vi "12.2-3 ParticleRemove.vi"() -> ()   [LabVIEW 2016]
doc: "This example shows how to use the Edge Tool in NI Vision. The Edge Tool finds edges (or sharp transitions in the pixels values) along a given line or ROI profile. The Edge Tool is a precursor function to many of the gauging and inspection tasks. For example, the location of the edges found along a line profile across an object can interpreted as the boundaries of the object whose dimensions have to be measured for a gauging application or the presence of a crack in the surface of an object for an inspection application."
uses:
  <vilib>/vision/NI_Vision_Development_Module.lvlib
panel:
  in  "Connectivity":bool
  in  "Filter":bool
  out "Src":T1(plugin-control)
  in  "Hexa Pixel?":bool
  in  "# of iterations":i32=20
  out "Dst":T1(plugin-control)
  in  "Stop":bool
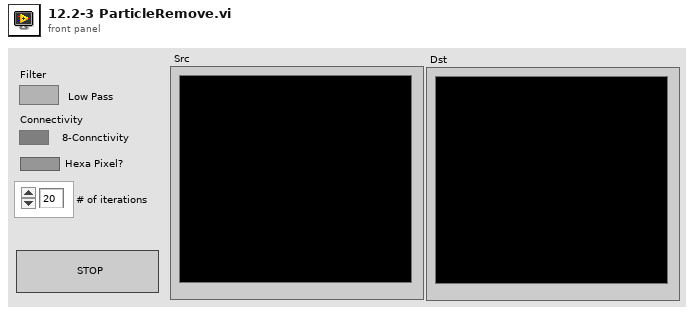
[diagram p1: front panel]
types:
  T1 = typedef "IMAQ Image.ctl" = refnum<image>
  T2 = cluster{"Connectivity":bool, "Hexa Pixel?":bool, "# of iterations":i32, "Filter":bool}
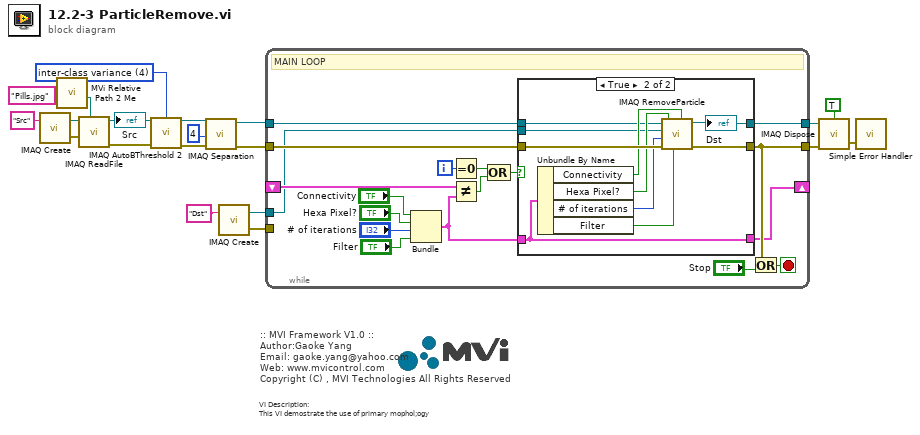
[diagram p0: block diagram]
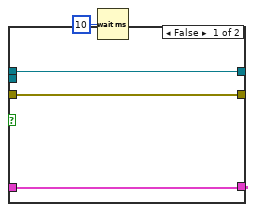
[diagram p2: hidden frame]
diagram:
  w9 = 4 items=["clustering", "entropy", "metric", "moments", "inter-class variance"] ("Method")
  # "VI Description:\nThis VI demostrate the use of primary mophol;ogy"
  # ":: MVI Framework V1.0 ::\nAuthor:Gaoke Yang\nEmail: gaoke.yang@yahoo.com\nWeb: www.mvicontrol.com\nCopyright (C) , MVI Technologies All Rights Reserved"
  n1 = call "IMAQ Create"("Image Name"="Src") -> ("New Image"=w19:T1, "error out"=w18:errorcluster)  [unwired: 4 in]
  n2 = call "MVi Relative Path 2 Me.vi"("Relative Path"="Pills.jpg" ("name or relative path")) -> ("Appended Dir"=w14:path)  [unwired: 5 in, 1 out]
  n3 = call "IMAQ ReadFile"("File Path"=w14, "error in (no error)"=w18, "Image"=w19) -> ("error out"=w8:errorcluster, "Image Out"=w7:T1)  [unwired: 4 in, 3 out]
  "Src" <- w7
  n4 = call "IMAQ AutoBThreshold 2"("Image Src"=w7, "Method (clustering)"=w9, "error in (no error)"=w8) -> ("Image Dst Out"=w3:T1, "error out"=w5:errorcluster)  [unwired: 5 in, 6 out]
  n5 = call "IMAQ Separation"("error in (no error)"=w5, "Nb of Erosion"=4, "Image Src"=w3) -> ("error out"=w4:errorcluster, "Image Dst Out"=w1:T1)  [unwired: 7 in]
  n6 = call "IMAQ Create"("Image Name"="Dst") -> ("New Image"=w11:T1, "error out"=w10:errorcluster)  [unwired: 4 in]
  n7 = while "MAIN LOOP" {
    tunnel: w1 -> [w37]
    tunnel: w4 -> [w38]
    tunnel: [w33] -> w17
    tunnel: [w34] -> w16
    shift-right: [w30] -> _
    shift-left: _ -> [w27]
    tunnel: w11 -> [w21]
    tunnel: w10 -> [_]
    i -> [w32]
    stop <- w35 stop-if-true
    # "MAIN LOOP"
    n8 = Bundle("Connectivity"="Connectivity", "Hexa Pixel?"="Hexa Pixel?", "# of iterations"="# of iterations", "Filter"="Filter") -> (w28:T2)  [unwired: 1 in]
    n9 = Equal To 0?(x=w32) -> (x = 0?=w29:bool)
    n10 = Not Equal?(x=w27, y=w28) -> (x != y?=w26:bool)
    n11 = Compound Arithmetic op=OR(w29, w26) -> (w31:bool)
    n12 = case shown="True" w31 {
      tunnel: w38 -> [w41 w51]
      tunnel: w37 -> [w42 w44]
      tunnel: [w42 w49] -> w34
      tunnel: [w41 w50] -> w33
      tunnel: [w39 w52] -> w30
      tunnel: w28 -> [w39 w52]
      tunnel: w21 -> [_ w43]
      frame False {
        n13 = Wait (ms)(milliseconds to wait=u32 10) -> ()  [unwired: 1 out]
      }
      frame True {
        n14 = Unbundle By Name(w52) -> ("Connectivity"=w48:bool, "Hexa Pixel?"=w47:bool, "# of iterations"=w46:i32, "Filter"=w45:bool)
        n15 = call "IMAQ RemoveParticle"("Connectivity 4/8 (8)"=w48, "Low Pass/High Pass (Low)"=w45, "Square/Hexa (Square)"=w47, "error in (no error)"=w51, "Number of Erosion"=w46, "Image Dst"=w43, "Image Src"=w44) -> ("error out"=w50:errorcluster, "Image Dst Out"=w49:T1)  [unwired: 3 in]
        "Dst" <- w49
      }
    }
    n16 = Or(x=w33, y="Stop") -> (x .or. y?=w35:bool)
  }
  n17 = call "IMAQ Dispose"("All Images? (No)"=TRUE, "Image"=w16, "error in (no error)"=w17) -> ("error out"=w13:errorcluster)  [unwired: 3 in]
  n18 = call <vilib>:"Simple Error Handler.vi"("error in (no error)"=w13) -> ()  [unwired: 4 in, 5 out]
